vi "Untitled 1.vi"() -> ()   [LabVIEW 2020]
uses:
  <vilib>/Analysis/baseanly.llb/Mean (DBL).vi
  <vilib>/Analysis/NI_AALBase.lvlib
  <vilib>/Analysis/NI_AALPro.lvlib
panel:
  out "电阻的伏安特性曲线图":cluster{"Y":dbl[], "Y":dbl[]}[](graph)
  in  "中途停止（左键长按）":bool
  in  "电压递增步长(V)":dbl
  in  "电压上限(V)":dbl
  out "数据":dbl[][](array[numeric])
  in  "标准电阻值（欧姆）":dbl
  in  "采集时间间隔":dbl[unit]
  in  "待测电阻值（欧姆）":dbl
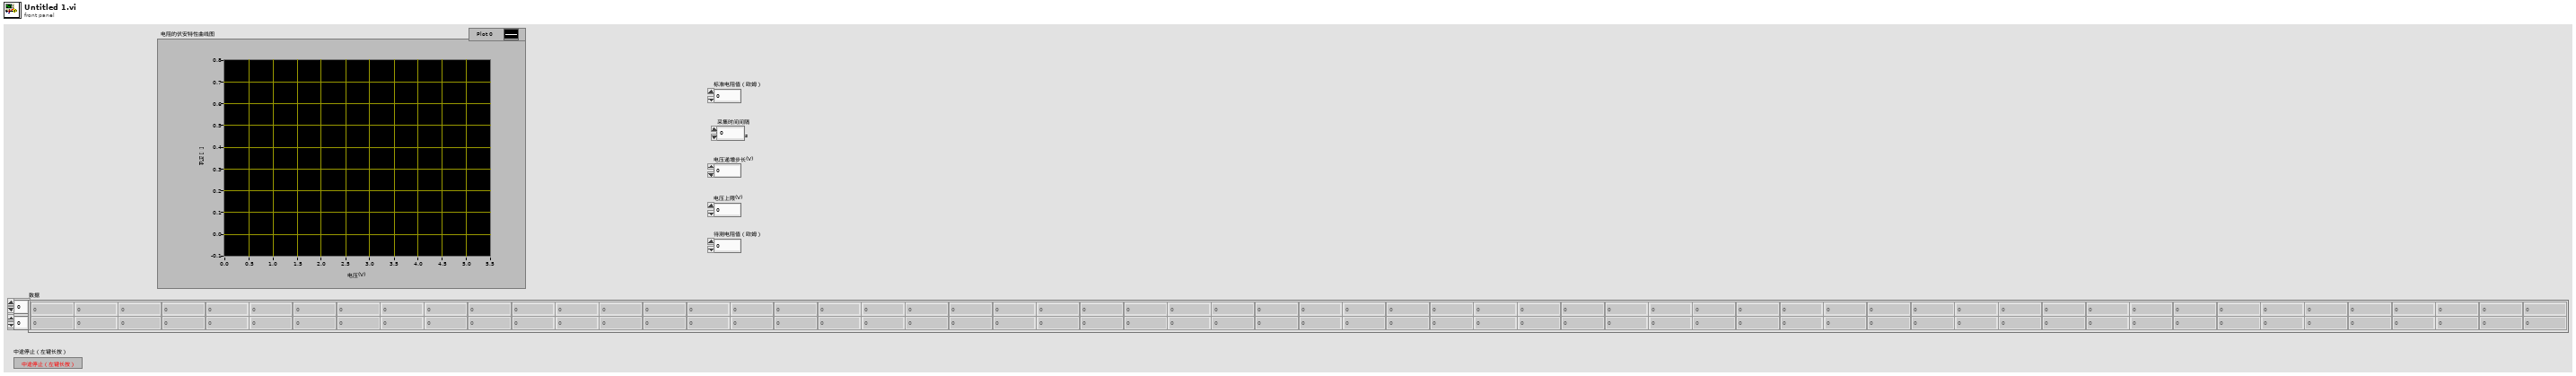
[diagram p1: front panel]
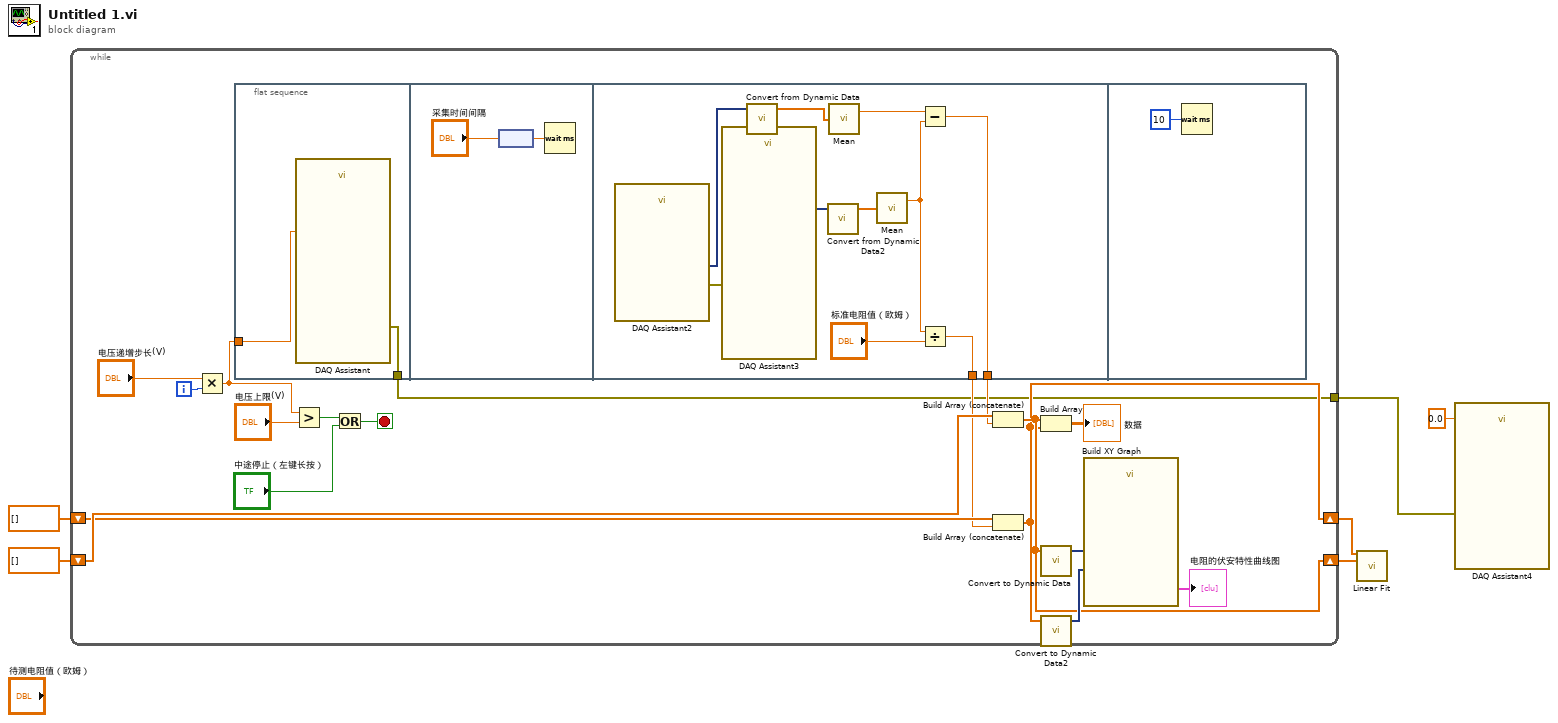
[diagram p0: block diagram]
diagram:
  n1 = while {
    shift-right: [w9] -> w4
    shift-left: dbl[] [] -> [w16]
    shift-right: [w8] -> w3
    shift-left: dbl[] [] -> [w15]
    tunnel: [w7] -> w1
    i -> [w22]
    stop <- w17 stop-if-true
    n2 = Multiply(x="电压递增步长(V)", y=w22) -> (x*y=w21:dbl)
    n3 = flat-sequence {
      tunnel: w21 -> [w26]
      tunnel: [w25] -> w7
      tunnel: [w30] -> w14
      tunnel: [w29] -> w13
      frame #0 {
        n4 = call "DAQ Assistant"("data"=w26) -> ("error out"=w25:errorcluster)  [unwired: 17 in, 1 out]
      }
      frame #1 {
        n5 = node("采集时间间隔") -> (w27:dbl)
        n6 = Wait (ms)(milliseconds to wait=w27) -> ()  [unwired: 1 out]
      }
      frame #2 {
        n7 = call "DAQ Assistant2"() -> ("data"=w37:dynamicdata, "error out"=w38:errorcluster)  [unwired: 17 in, 1 out]
        n8 = call "DAQ Assistant3"("error in"=w38) -> ("data"=w35:dynamicdata)  [unwired: 16 in, 2 out]
        n9 = call "Convert from Dynamic Data"("Dynamic Data Type"=w37) -> ("Array"=w36:dbl[])  [unwired: 3 in]
        n10 = call "Convert from Dynamic Data2"("Dynamic Data Type"=w35) -> ("Array"=w34:dbl[])  [unwired: 3 in]
        n11 = call-poly <vilib>:"Mean.vi"("X"=w36) -> ("mean"=w33:dbl)  [unwired: 1 out]
        n12 = call-poly <vilib>:"Mean.vi"("X"=w34) -> ("mean"=w32:dbl)  [unwired: 1 out]
        n13 = Subtract(x=w33, y=w32) -> (x-y=w30:dbl)
        n14 = Divide(x=w32, y="标准电阻值（欧姆）") -> (x/y=w29:dbl)
      }
      frame #3 {
        n15 = Wait (ms)(milliseconds to wait=10) -> ()  [unwired: 1 out]
      }
    }
    n16 = Greater?(x=w21, y="电压上限(V)") -> (0:w19:bool)
    n17 = Or(x=w19, y="中途停止（左键长按）") -> (x .or. y?=w17:bool)
    n18 = Build Array (concatenate)(w16, w14) -> (w9:dbl[])
    n19 = Build Array (concatenate)(w15, w13) -> (w8:dbl[])
    n20 = Build Array(w9, w8) -> (→"数据":dbl[][])
    n21 = call "Convert to Dynamic Data"("Array"=w9) -> ("Dynamic Data Type"=w11:dynamicdata)  [unwired: 3 in]
    n22 = call "Convert to Dynamic Data2"("Array"=w8) -> ("Dynamic Data Type"=w10:dynamicdata)  [unwired: 3 in]
    n23 = call "Build XY Graph"("Y Input"=w10, "X Input"=w11) -> ("XY Graph"=→"电阻的伏安特性曲线图":cluster{"X":dbl[], "Y":dbl[]}[])  [unwired: 8 in, 1 out]
  }
  n24 = call <vilib>:"Linear Fit.vi"("Y"=w3, "X"=w4) -> ()  [unwired: 9 in, 5 out]
  n25 = call "DAQ Assistant4"("data"=0.0, "error in"=w1) -> ()  [unwired: 16 in, 2 out]
